vi "Write MIDI dwMsg.vi"(8 "channel":u8, 9 "MIDI_event":u8, 10 "lo_byte":u8, 11 "hi_byte":u8) -> (2 "event_dwMsg":u32)   [LabVIEW 8.6]
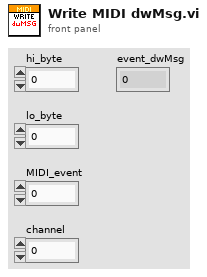
[diagram p1: front panel]
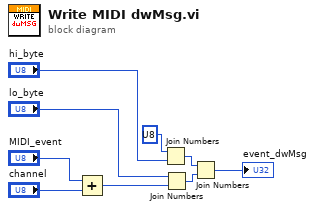
[diagram p0: block diagram]
diagram:
  n1 = Add(x="MIDI_event", y="channel") -> (x+y=w5:u8)
  n2 = Join Numbers(hi=u8 ?, lo="hi_byte") -> ((hi.lo)=w2:u16)
  n3 = Join Numbers(hi="lo_byte", lo=w5) -> ((hi.lo)=w1:u16)
  n4 = Join Numbers(hi=w2, lo=w1) -> ((hi.lo)=→"event_dwMsg":u32)
